vi "GoTo Tangent.vi"(4 "Passe":bool, 6 "Cone de chute":dbl=0.55 format="%#_13g", 7 "IA State Input in":T2, 8 "distance between ball and robot":dbl=250.0 format="%#_13g", 9 "Ball":dbl[](array[numeric])=[-1986.6092529296875, -3009.6396484375], 10 "Target":dbl[](array[numeric]), 11 "R":dbl[](array[numeric])=[-2840.578369140625, -1536.7857666015625, -1.0371381044387817]) -> (1 "Destination":dbl[](array[numeric]), 2 "Output\nVelocity":dbl[](array[numeric]) format="%.2f")   [LabVIEW 2018]
uses:
  Core/AI Input.ctl
  Core/AI Robot.ctl
  Intel/Functions Enum.ctl
  Intel/AttackerStates.ctl
  Path Planning/RRT/PathDests.ctl
  Path Planning/RRT/PathDest.ctl
  Core/AI Ball.ctl
  Core/Field Size.ctl
  Core/AI Judge.ctl
  Intel/Command Enum.ctl
  Util/Events/Events.ctl
  <vilib>/Analysis/coordinate.llb/Angle Range (Degree).ctl
  <vilib>/Analysis/coordinate.llb/Wrap Angle (scalar).vi
  <vilib>/Analysis/coordinate.llb/2D Cartesian Coordinate Rotation (Scalar).vi
  <vilib>/Analysis/NI_AALPro.lvlib
  <vilib>/Analysis/NI_AAL_Angle.lvlib
panel:
  in  "f":dbl[](array[numeric])=[0.0, 0.0, 0.0]
  in  "mag force\neps":dbl
  in  "angle range":T1=1 items=["none", "-180 to 180 (-pi to pi)", "0 to 360 (0 to 2pi)"]
  out "Waveform Chart 2":dbl[][](graph)
  out "Robot":dbl[](array[numeric])=[-2840.578369140625, -1536.7857666015625, -1.0371381044387817]
  out "Waveform Chart":dbl[][](graph)
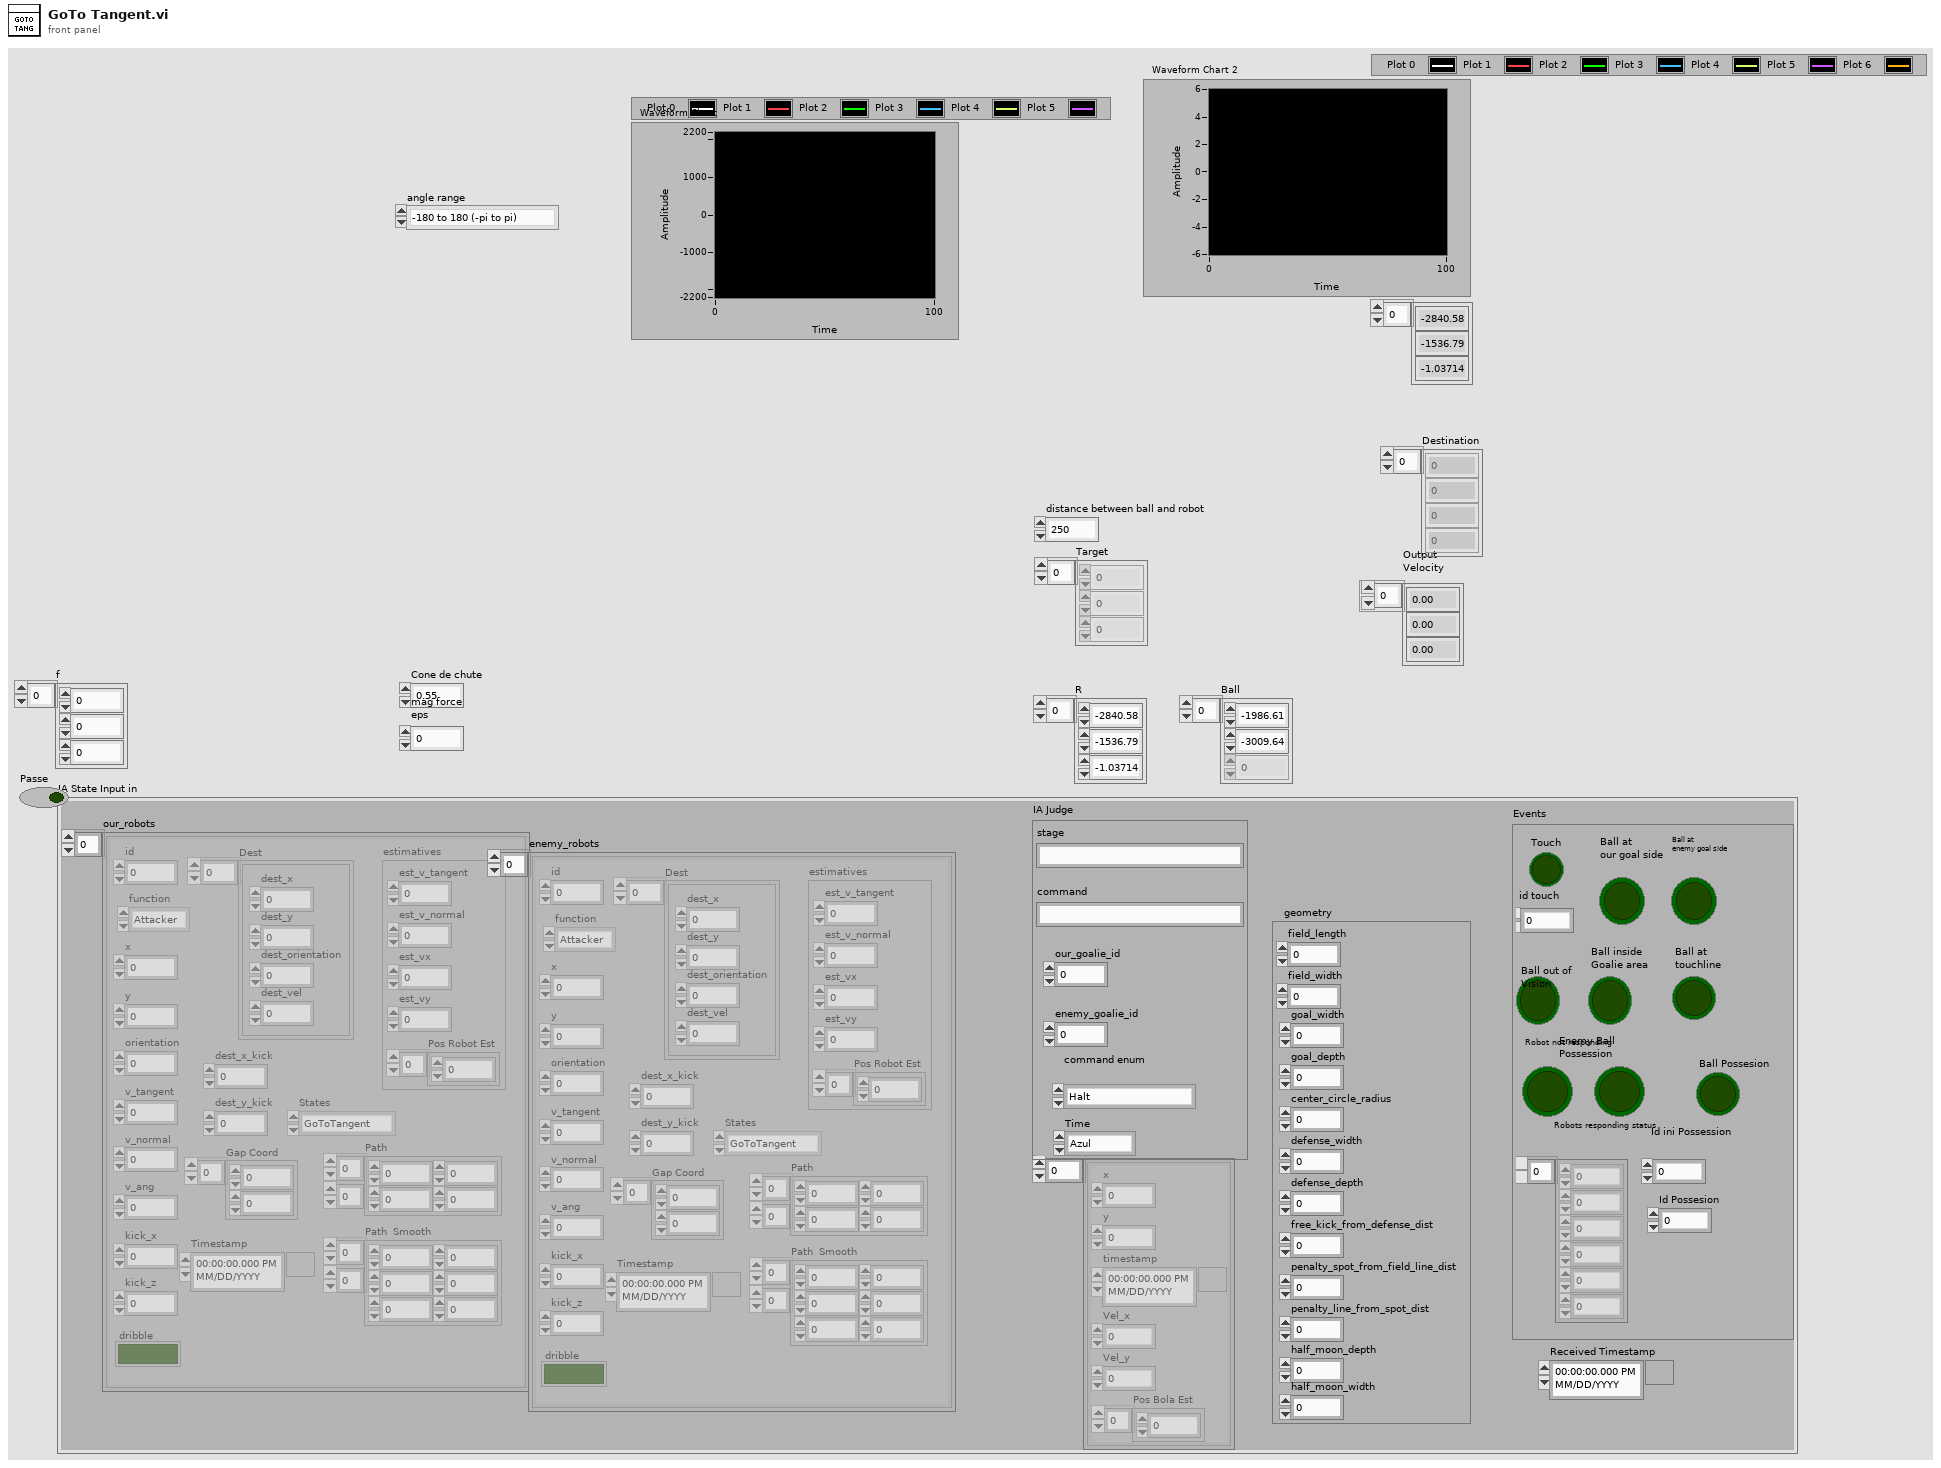
[diagram p1: front panel]
types:
  T1 = typedef "NI_AAL_Angle.lvlib/Angle Range (Degree).ctl" = u16
  T2 = typedef "AI Input.ctl" = cluster{"our_robots":T3[], "enemy_robots":T3[], "balls":T8[], "geometry":T9, "IA Judge":T10, "Received Timestamp":timestamp, "Events":T12}
  T3 = typedef "AI Robot.ctl" = cluster{"id":u32, "function":T4, "x":dbl, "y":dbl, "orientation":dbl, "v_tangent":dbl, "v_normal":dbl, "v_ang":dbl, "kick_x":dbl, "kick_z":dbl, "dribble":bool, "Timestamp":timestamp, "estimatives":cluster{"est_v_tangent":dbl, "est_v_normal":dbl, "est_vx":dbl, "est_vy":dbl, "Pos Robot Est":dbl[]}, "dest_x_kick":dbl, "dest_y_kick":dbl, "Gap Coord":dbl[], "States":T5, "Path ":dbl[][], "Path  Smooth":dbl[][], "Dest":T6}
  T4 = typedef "Functions Enum.ctl" = enum16{"Attacker", "Goalie", "Defender", "Striker", "Goto 0", "Dummy", "Kicker", "ZigZag"}
  T5 = typedef "AttackerStates.ctl" = enum16{"Pass", "GoToTangent", "BallGetting", "GoToKick", "Rotate anti-clockwise", "Rotate Clockwise", ""}
  T6 = typedef "PathDests.ctl" = T7[]
  T7 = typedef "PathDest.ctl" = cluster{"dest_x":dbl, "dest_y":dbl, "dest_orientation":dbl, "dest_vel":dbl}
  T8 = typedef "AI Ball.ctl" = cluster{"x":dbl, "y":dbl, "timestamp":timestamp, "Vel_x":dbl, "Vel_y":dbl, "Pos Bola Est":dbl[]}
  T9 = typedef "Field Size.ctl" = cluster{"field_length":u32, "field_width":u32, "goal_width":u32, "goal_depth":u32, "center_circle_radius":u32, "defense_width":u32, "defense_depth":u32, "free_kick_from_defense_dist":u32, "penalty_spot_from_field_line_dist":u32, "penalty_line_from_spot_dist":u32, "half_moon_depth":u32, "half_moon_width":u32}
  T10 = typedef "AI Judge.ctl" = cluster{"stage":string, "command":string, "our_goalie_id":dbl, "enemy_goalie_id":dbl, "command enum":T11, "Time":enum16{"Azul", "Amarelo"}}
  T11 = typedef "Command Enum.ctl" = enum16{"Halt", "Stop", "Force Start", "PKA Normal Start", "Prepare Kickoff Ally", "PKE Normal Start", "Prepare Kickoff Enemy", "Prepare Penalty Ally", "PPA Normal Start", "Prepare Penalty Enemy", "PPE Normal Start", "Ball Placement Enemy Up", "Ball Placement Enemy Down", "Ball Placement Ally Up", "Ball Placement Ally Mid", "Ball Placement Ally Down", "Indirect Free Enemy", "Indirect Free Ally", "Timeout Enemy", "Timeout Ally", "Goal Enemy", "Goal Ally", "Normal Half Time", "Extra Time Break", "Extra Half Time", "None", "Post Game"}
  T12 = typedef "Events.ctl" = cluster{"Touch":bool, "id touch":dbl, "Ball out of \nVision":bool, "Ball inside \nGoalie area":bool, "Robot not responding":bool, "Robots responding status":dbl[], "Enemy Ball \nPossession":bool, "Id ini Possession":dbl, "Ball Possesion":bool, "Id Possesion":dbl, "Ball at\nour goal side":bool, "Ball at\ntouchline":bool, "Ball at\nenemy goal side":bool}
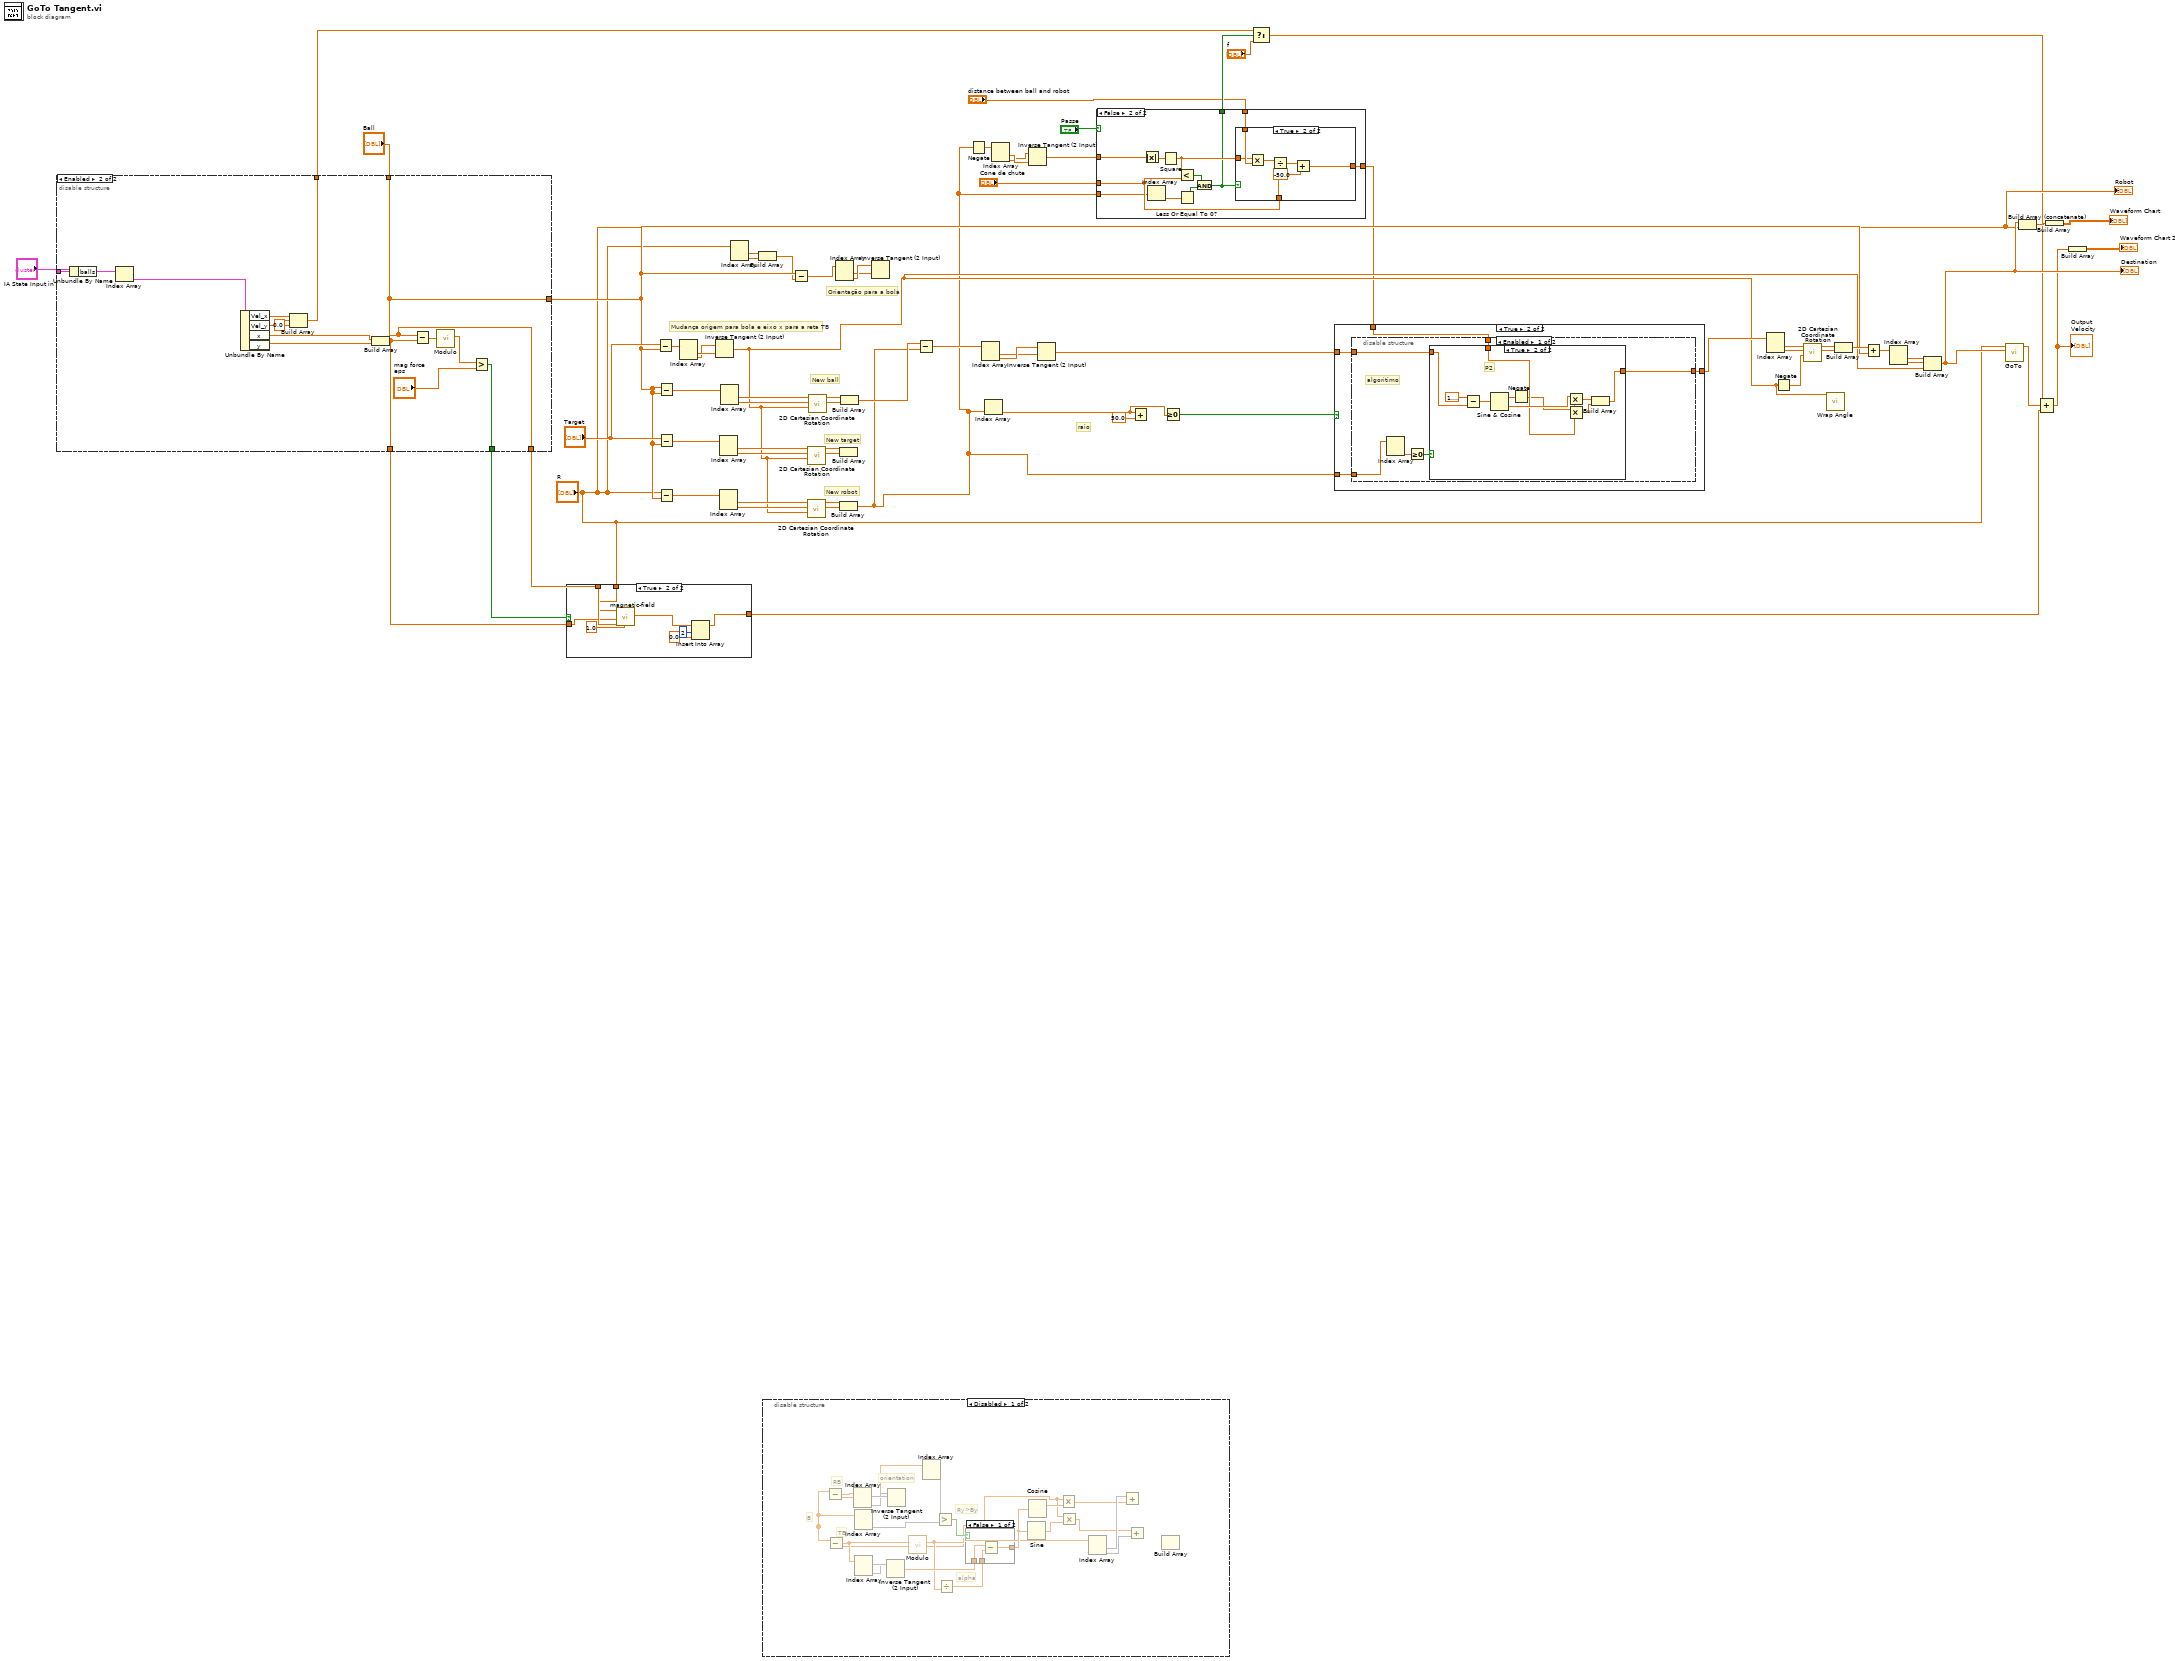
[diagram p0: block diagram]
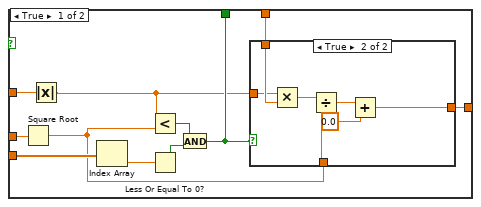
[diagram p2: hidden frame]
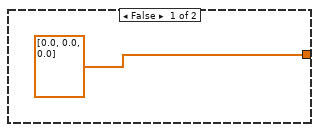
[diagram p5: hidden frame]
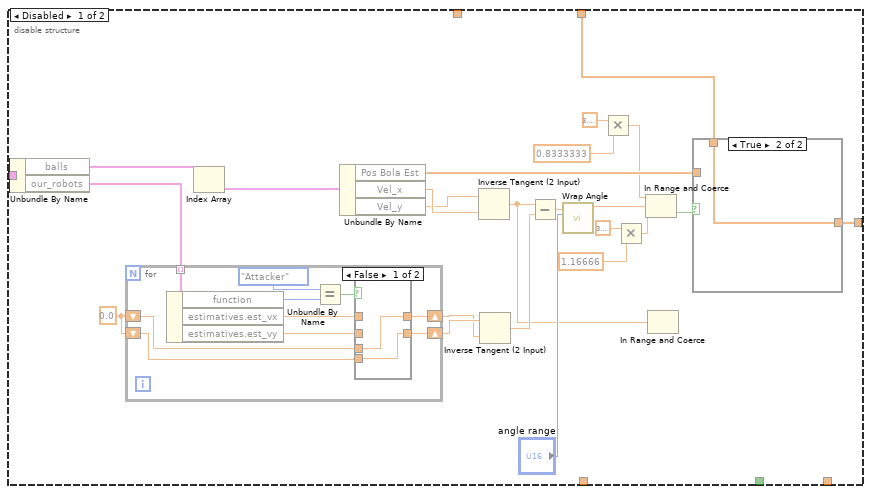
[diagram p6: hidden frame]
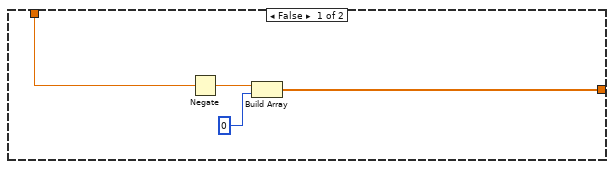
[diagram p9: hidden frame]
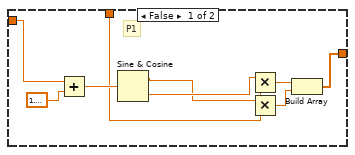
[diagram p10: hidden frame]
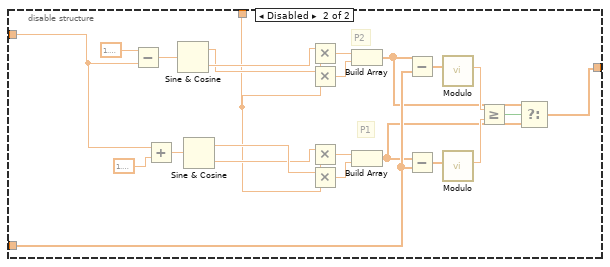
[diagram p11: hidden frame]
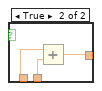
[diagram p12: hidden frame]
diagram:
  # "raio"
  # "New ball"
  # "New target"
  # "New robot"
  # "Orientação para a bola"
  # "Mudança origem para bola e eixo x para a reta TB"
  n1 = disable-structure shown="Enabled" {
    disable-tunnel: [w95 w116] -> w30
    disable-tunnel: "IA State Input in" -> [w94 w125]
    disable-tunnel: "Ball" -> [w72 w116]
    disable-tunnel: [_ w117] -> w16
    disable-tunnel: [_ w116] -> w15
    disable-tunnel: [_ w115] -> w14
    disable-tunnel: [_ w113] -> w9
    frame Disabled {
      w90 = 0.0 ("est_vx")
      n2 = Unbundle By Name(w94) -> ("balls"=w93:T8[], "our_robots"=w91:T3[])
      n3 = for {
        tunnel: w91 -> [w105] mode=indexing
        shift-right: [w101] -> w87
        shift-left: w90 -> [w97]
        shift-right: [w98] -> w88
        shift-left: w90 -> [w96]
        n4 = Unbundle By Name(w105) -> ("function"=w103:T4, "estimatives.est_vx"=w100:dbl, "estimatives.est_vy"=w99:dbl)
        n5 = Equal?(x=Functions_Enum."Attacker" ("function"), y=w103) -> (x = y?=w104:bool)
        n6 = case shown="False" w104 {
          tunnel: [w107 w109] -> w101
          tunnel: w100 -> [_ w109]
          tunnel: w99 -> [_ w108]
          tunnel: [w106 w108] -> w98
          tunnel: w97 -> [w107 _]
          tunnel: w96 -> [w106 _]
          frame False {
          }
          frame True {
          }
        }
      }
      n7 = Index Array(array=w93) -> (element=w92:T8)  [unwired: 1 in]
      n8 = Unbundle By Name(w92) -> ("Pos Bola Est"=w89:dbl[], "Vel_x"=w86:dbl, "Vel_y"=w85:dbl)
      n9 = Inverse Tangent (2 Input)(1:w86, 2:w85) -> (0:w73:dbl)
      n10 = Inverse Tangent (2 Input)(1:w87, 2:w88) -> (0:w84:dbl)
      n11 = Subtract(x=w73, y=w84) -> (x-y=w82:dbl)
      n12 = call-poly <vilib>:"Wrap Angle.vi"("angle range"="angle range", "angle in"=w82) -> ("angle out"=w78:dbl)  [unwired: 8 in, 1 out]
      n13 = Multiply(x=3.141592653589793, y=0.8333333) -> (x*y=w75:dbl)
      n14 = Multiply(x=3.141592653589793, y=1.16666) -> (x*y=w81:dbl)
      n15 = In Range and Coerce(upper limit=w75, x=w78, lower limit=w81) -> (In Range?=w74:bool)  [unwired: 1 out]
      n16 = In Range and Coerce(x=w73) -> ()  [unwired: 2 in, 2 out]
      n17 = case shown="True" w74 {
        tunnel: [_ w110] -> w95
        tunnel: w89 -> [_ _]
        tunnel: w72 -> [_ w110]
        frame False {
        }
        frame True {
        }
      }
    }
    frame Enabled {
      n18 = Unbundle By Name(w125) -> ("balls"=w123:T8[])
      n19 = Index Array(array=w123) -> (element=w124:T8)  [unwired: 1 in]
      n20 = Unbundle By Name(w124) -> ("Vel_x"=w114:dbl, "Vel_y"=w112:dbl, "x"=w122:dbl, "y"=w121:dbl)
      n21 = Build Array(w114, w112, 0.0 ("element")) -> (w113:dbl[])
      n22 = Build Array(w122, w121) -> (w115:dbl[])
      n23 = Subtract(x=w116, y=w115) -> (x-y=w120:dbl[])
      n24 = call "Modulo.vi"("2D vector"=w120) -> ("Modulo"=w119:dbl)  [unwired: 10 in]
      n25 = Greater?(x=w119, y="mag force\neps") -> (0:w117:bool)
    }
  }
  n26 = case shown="True" w16 {
    tunnel: w15 -> [_ w133]
    tunnel: w14 -> [_ w132]
    tunnel: "R" -> [_ w131]
    tunnel: [dbl[] [0.0, 0.0, 0.0] ("magnetic force") w128] -> w12
    frame False {
    }
    frame True {
      n27 = call "magnetic-field.vi"("max force"=1.0, "goal pos"=w133, "enemy pos"=w132, "ally pos"=w131) -> ("magnetic force"=w129:dbl[])  [unwired: 7 in]
      n28 = Insert Into Array(array=w129, index=2, new element=0.0 ("new element/subarray")) -> (w128:dbl[])
    }
  }
  n29 = Subtract(x="Target", y=w30) -> (x-y=w62:dbl[])
  n30 = Subtract(x=w30, y=w30) -> (x-y=w69:dbl[])
  n31 = Subtract(x="Target", y=w30) -> (x-y=w66:dbl[])
  n32 = Subtract(x="R", y=w30) -> (x-y=w63:dbl[])
  n33 = Index Array(array=w62) -> (element #1=w61:dbl, element #2=w60:dbl)  [unwired: 2 in]
  n34 = Inverse Tangent (2 Input)(1:w61, 2:w60) -> (0:w24:dbl)
  n35 = Index Array(array=w63) -> (element #1=w65:dbl, element #2=w64:dbl)  [unwired: 2 in]
  n36 = Index Array(array=w66) -> (element #1=w68:dbl, element #2=w67:dbl)  [unwired: 2 in]
  n37 = Index Array(array=w69) -> (element #1=w71:dbl, element #2=w70:dbl)  [unwired: 2 in]
  n38 = Index Array(array="R") -> (element #1=w29:dbl, element #2=w28:dbl)  [unwired: 2 in]
  n39 = Build Array(w29, w28) -> (w27:dbl[])
  n40 = disable-structure shown="Disabled" {
    frame Disabled {
      # "Ry>By"
      # "orientation"
      # "RB"
      # "alpha"
      # "TB"
      # "B"
      n41 = Index Array() -> (array=w140:dbl[], element #2=w146)  [unwired: 2 in, 1 out]
      n42 = Index Array() -> (array=w136:dbl[], element #2=w147)  [unwired: 2 in, 1 out]
      n43 = Subtract(x=w140, y=w136) -> (x-y=w154:dbl)
      n44 = Index Array(array=w154) -> (element #1=w156, element #2=w155)  [unwired: 2 in]
      n45 = Inverse Tangent (2 Input)(1:w156, 2:w155) -> (0:w153:dbl)
      n46 = Greater?(x=w147, y=w146) -> (0:w145:bool)
      n47 = Index Array() -> (array=w135:dbl[], element #1=w143, element #2=w138)  [unwired: 2 in]
      n48 = Subtract(x=w140, y=w135) -> (x-y=w158:dbl)
      n49 = Index Array(array=w158) -> (element #1=w160, element #2=w159)  [unwired: 2 in]
      n50 = Inverse Tangent (2 Input)(1:w160, 2:w159) -> (0:w152:dbl)
      n51 = call "Modulo.vi"("2D vector"=w158) -> ("Modulo"=w144:dbl)  [unwired: 10 in]
      n52 = Divide(y=w144) -> (x=w157:dbl, x/y=w151:dbl)
      n53 = case shown="False" w145 {
        tunnel: w152 -> [w162 w166]
        tunnel: w151 -> [w163 w165]
        tunnel: [w161 w164] -> w150
        frame False {
          n54 = Subtract(x=w162, y=w163) -> (x-y=w161:dbl)
        }
        frame True {
          n55 = Add(x=w166, y=w165) -> (x+y=w164:dbl)
        }
      }
      n56 = Sine(x=w150) -> (sin(x)=w148:dbl)
      n57 = Cosine(x=w150) -> (cos(x)=w149:dbl)
      n58 = Multiply(x=w144, y=w149) -> (x*y=w142:dbl)
      n59 = Multiply(x=w144, y=w148) -> (x*y=w139:dbl)
      n60 = Add(x=w143, y=w142) -> (x+y=w141:dbl)
      n61 = Add(x=w139, y=w138) -> (x+y=w137:dbl)
      n62 = Build Array() -> ()  [unwired: 3 in, 1 out]
    }
    frame Enabled {
    }
  }
  n63 = Subtract(x=w30, y=w27) -> (x-y=w42:dbl[])
  n64 = call-poly <vilib>:"2D Cartesian Coordinate Rotation.vi"("theta"=w24, "y"=w64, "x"=w65) -> ("y out"=w54:dbl, "x out"=w55:dbl)  [unwired: 6 in, 1 out]
  n65 = call-poly <vilib>:"2D Cartesian Coordinate Rotation.vi"("theta"=w24, "y"=w67, "x"=w68) -> ("y out"=w58:dbl, "x out"=w59:dbl)  [unwired: 6 in, 1 out]
  n66 = call-poly <vilib>:"2D Cartesian Coordinate Rotation.vi"("theta"=w24, "y"=w70, "x"=w71) -> ("y out"=w56:dbl, "x out"=w57:dbl)  [unwired: 6 in, 1 out]
  n67 = Index Array(array=w42) -> (element #1=w43:dbl, element #2=w44:dbl)  [unwired: 2 in]
  n68 = Build Array(w55, w54) -> (w17:dbl[])
  n69 = Build Array(w59, w58) -> ()  [unwired: 1 out]
  n70 = Build Array(w57, w56) -> (w37:dbl[])
  n71 = Inverse Tangent (2 Input)(1:w43, 2:w44) -> ()  [unwired: 1 out]
  n72 = Subtract(x=w37, y=w17) -> (x-y=w51:dbl[])
  n73 = Negate(x=w17) -> (-x=w23:dbl[])
  n74 = Index Array(array=w51) -> (element #1=w52:dbl, element #2=w53:dbl)  [unwired: 2 in]
  n75 = Index Array(array=w17) -> (element=w2:dbl)  [unwired: 1 in]
  n76 = Index Array(array=w23) -> (element #1=w22:dbl, element #2=w21:dbl)  [unwired: 2 in]
  n77 = Inverse Tangent (2 Input)(1:w22, 2:w21) -> (0:w20:dbl)
  n78 = Inverse Tangent (2 Input)(1:w52, 2:w53) -> (0:w38:dbl)
  n79 = case shown="False" "Passe" {
    tunnel: w20 -> [w177 w196]
    tunnel: "Cone de chute" -> [w169 w195]
    tunnel: [w176 w194] -> w18
    tunnel: "distance between ball and robot" -> [w175 w193]
    tunnel: w17 -> [w174 w190]
    tunnel: [w170 w186] -> w8
    frame True {
      n80 = Square Root(x=w169) -> (sqrt(x)=w167:dbl)
      n81 = Absolute Value(x=w177) -> (abs(x)=w168:dbl)
      n82 = Index Array(array=w174) -> (element=w173:dbl)  [unwired: 1 in]
      n83 = Less?(x=w168, y=w167) -> (x < y?=w172:bool)
      n84 = Less Or Equal To 0?(x=w173) -> (x <= 0?=w171:bool)
      n85 = And(x=w172, y=w171) -> (x .and. y?=w170:bool)
      n86 = case shown="True" w170 {
        tunnel: w167 -> [_ w183]
        tunnel: [w178 w182] -> w176
        tunnel: w175 -> [w178 w181]
        tunnel: w168 -> [_ w180]
        frame False {
        }
        frame True {
          n87 = Multiply(x=w180, y=w181) -> (x*y=w185:dbl)
          n88 = Divide(x=w185, y=w183) -> (x/y=w184:dbl)
          n89 = Add(x=w184, y=0.0) -> (x+y=w182:dbl)
        }
      }
    }
    frame False {
      n90 = Absolute Value(x=w196) -> (abs(x)=w192:dbl)
      n91 = Index Array(array=w190) -> (element=w189:dbl)  [unwired: 1 in]
      n92 = Square(x=w192) -> (x^2=w191:dbl)
      n93 = Less?(x=w191, y=w195) -> (x < y?=w188:bool)
      n94 = Less Or Equal To 0?(x=w189) -> (x <= 0?=w187:bool)
      n95 = And(x=w188, y=w187) -> (x .and. y?=w186:bool)
      n96 = case shown="True" w186 {
        tunnel: w195 -> [_ w202]
        tunnel: [w197 w201] -> w194
        tunnel: w193 -> [w197 w200]
        tunnel: w191 -> [_ w199]
        frame False {
        }
        frame True {
          n97 = Multiply(x=w199, y=w200) -> (x*y=w204:dbl)
          n98 = Divide(x=w204, y=w202) -> (x/y=w203:dbl)
          n99 = Add(x=w203, y=-50.0) -> (x+y=w201:dbl)
        }
      }
    }
  }
  n100 = Add(x=w2, y=50.0) -> ()  [unwired: 1 out]
  n101 = Greater Or Equal To 0?(x=w2) -> (x >= 0?=w3:bool)
  n102 = Select(t=w9, s=w8, f="f") -> (s? t:f=w6:dbl[])
  n103 = case shown="True" w3 {
    tunnel: w38 -> [_ w212]
    tunnel: [w207 w211] -> w46
    tunnel: w17 -> [_ w210]
    tunnel: w18 -> [w205 w209]
    frame False {
      n104 = Negate(x=w205) -> (-x=w206:dbl)
      n105 = Build Array(w206, 0 ("index")) -> (w207:dbl[])
    }
    frame True {
      n106 = disable-structure shown="Enabled" {
        disable-tunnel: w212 -> [w217 w248]
        disable-tunnel: [w216 w240] -> w211
        disable-tunnel: w210 -> [w214 w246]
        disable-tunnel: w209 -> [w213 w249]
        frame Enabled {
          # "algoritimo"
          n107 = Index Array(array=w214) -> (element #2=w218:dbl)  [unwired: 2 in, 1 out]
          n108 = Greater Or Equal To 0?(x=w218) -> (x >= 0?=w215:bool)
          n109 = case shown="True" w215 {
            tunnel: w217 -> [w222 w231]
            tunnel: [w224 w234] -> w216
            tunnel: w213 -> [w220 w230]
            frame False {
              # "P1"
              n110 = Add(x=w222, y=1.5707963267948966) -> (x+y=w223:dbl)
              n111 = Sine & Cosine(0:w223) -> (1:w219:dbl, 2:w225:dbl)
              n112 = Multiply(x=w225, y=w220) -> (x*y=w227:dbl)
              n113 = Multiply(x=w219, y=w220) -> (x*y=w226:dbl)
              n114 = Build Array(w227, w226) -> (w224:dbl[])
            }
            frame True {
              # "P2"
              n115 = Subtract(x=1.5707963267948966, y=w231) -> (x-y=w233:dbl)
              n116 = Sine & Cosine(0:w233) -> (1:w229:dbl, 2:w237:dbl)
              n117 = Negate(x=w229) -> (-x=w228:dbl)
              n118 = Multiply(x=w237, y=w230) -> (x*y=w235:dbl)
              n119 = Multiply(x=w228, y=w230) -> (x*y=w236:dbl)
              n120 = Build Array(w235, w236) -> (w234:dbl[])
            }
          }
        }
        frame Disabled {
          # "P1"
          # "P2"
          n121 = Subtract(x=1.5707963267948966, y=w248) -> (x-y=w256:dbl)
          n122 = Add(x=w248, y=1.5707963267948966) -> (x+y=w251:dbl)
          n123 = Sine & Cosine(0:w256) -> (1:w259:dbl, 2:w260:dbl)
          n124 = Sine & Cosine(0:w251) -> (1:w253:dbl, 2:w252:dbl)
          n125 = Multiply(x=w260, y=w249) -> (x*y=w257:dbl)
          n126 = Multiply(x=w259, y=w249) -> (x*y=w258:dbl)
          n127 = Multiply(x=w252, y=w249) -> (x*y=w255:dbl)
          n128 = Multiply(x=w253, y=w249) -> (x*y=w254:dbl)
          n129 = Build Array(w257, w258) -> (w239:dbl[])
          n130 = Build Array(w255, w254) -> (w238:dbl[])
          n131 = Subtract(x=w239, y=w246) -> (x-y=w242:dbl[])
          n132 = Subtract(x=w238, y=w246) -> (x-y=w241:dbl[])
          n133 = call "Modulo.vi"("2D vector"=w242) -> ("Modulo"=w245:dbl)  [unwired: 10 in]
          n134 = call "Modulo.vi"("2D vector"=w241) -> ("Modulo"=w244:dbl)  [unwired: 10 in]
          n135 = Greater Or Equal?(x=w245, y=w244) -> (x >= y?=w243:bool)
          n136 = Select(t=w239, s=w243, f=w238) -> (s? t:f=w240:dbl[])
        }
      }
    }
  }
  n137 = Index Array(array=w46) -> (element #1=w50:dbl, element #2=w49:dbl)  [unwired: 2 in]
  n138 = Negate(x=w24) -> (-x=w35:dbl)
  n139 = call-poly <vilib>:"2D Cartesian Coordinate Rotation.vi"("theta"=w35, "y"=w49, "x"=w50) -> ("y out"=w47:dbl, "x out"=w48:dbl)  [unwired: 6 in, 1 out]
  n140 = call-poly <vilib>:"Wrap Angle.vi"("angle in"=w24) -> ()  [unwired: 9 in, 2 out]
  n141 = Build Array(w48, w47) -> (w45:dbl[])
  n142 = Add(x=w45, y=w30) -> (x+y=w41:dbl[])
  n143 = Index Array(array=w41) -> (element #1=w40:dbl, element #2=w39:dbl)  [unwired: 2 in]
  n144 = Build Array(w40, w39, w24) -> (w36:dbl[])
  "Destination" <- w36
  n145 = call "GoTo.vi"("Target"=w36, "Position"="R") -> ("Output\nVelocity"=w11:dbl[])  [unwired: 8 in, 1 out]
  n146 = Build Array (concatenate)(w36, "R") -> (w34:dbl[])
  n147 = Compound Arithmetic op=ADD(w6, w11, w12) -> (w10:dbl[])
  "Output\nVelocity" <- w10
  n148 = Build Array(w34) -> (→"Waveform Chart":dbl[][])
  n149 = Build Array(w10) -> (→"Waveform Chart 2":dbl[][])
  "Robot" <- "R"
